vi "Alter Table Name.vi"(8 "error in":errorcluster, 9 "New table name":string, 10 "Existing Table name":string, 11 "Data.PG":refnum<class "LV-Data.PGSQL.lvclass">) -> (0 "error out":errorcluster, 2 "SQL":string, 3 "Data.PG out":refnum<class "LV-Data.PGSQL.lvclass">)   [LabVIEW 2016, in "LV-Data.PGSQL.lvclass"]
uses:
  LV-Data.PGSQL.lvclass
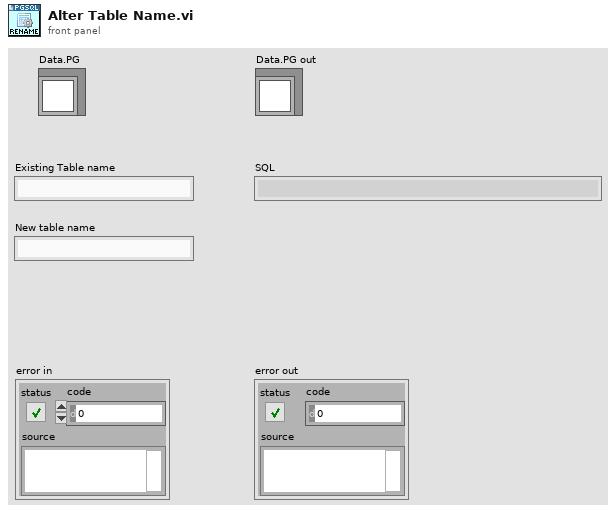
[diagram p1: front panel]
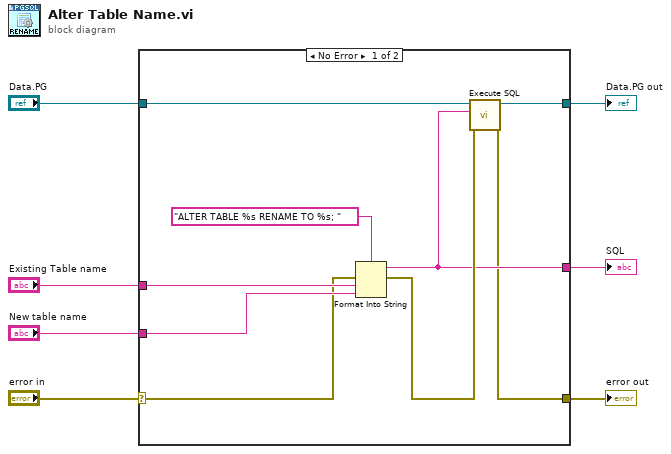
[diagram p0: block diagram]
diagram:
  n1 = case shown="No Error" "error in" {
    selector: "error in" -> [w8 w17]
    tunnel: "Existing Table name" -> [w15 _]
    tunnel: "New table name" -> [w14 _]
    tunnel: [w12 _] -> w5
    tunnel: [w11 w17] -> w4
    tunnel: "Data.PG" -> [w10 w18]
    tunnel: [w9 w18] -> w2
    frame No Error {
      n2 = Format Into String(format string="ALTER TABLE %s RENAME TO %s; ", error in=w8, w15, w14) -> (resulting string=w12:string, error out=w13:errorcluster)  [unwired: 1 in]
      n3 = call "Execute SQL.vi"("error in"=w13, "SQL"=w12, "Data.PG"=w10) -> ("error out"=w11:errorcluster, "Data.PG out"=w9:refnum<class "LV-Data.PGSQL.lvclass">)  [unwired: 6 in, 1 out]
    }
    frame Error {
    }
  }
  "SQL" <- w5
  "error out" <- w4
  "Data.PG out" <- w2
